vi "CMC-Random_Number_Alarms.vi"() -> ()   [LabVIEW 2010]
panel:
  out "Ok":bool
  out "Low Alarm":bool
  out "High Alarm":bool
  in  "Low Alarm":dbl=0.05 min=0.05 max=0.45
  in  "High Alarm":dbl=0.65 min=0.65 max=0.95 format="%#.2g"
  out "number(0 to 1)":dbl(slide) scale=0.0..1.0
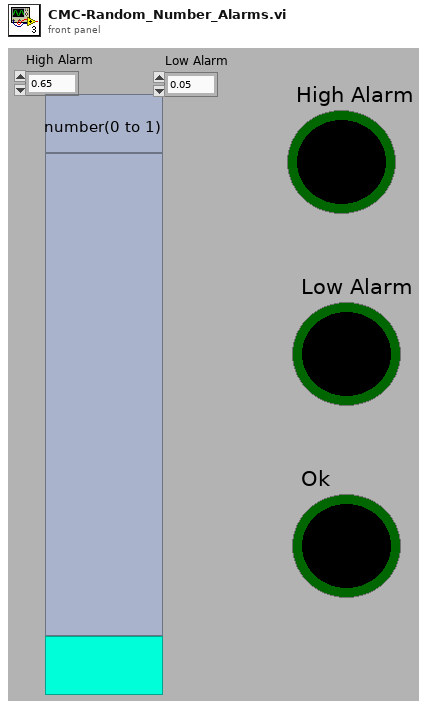
[diagram p1: front panel]
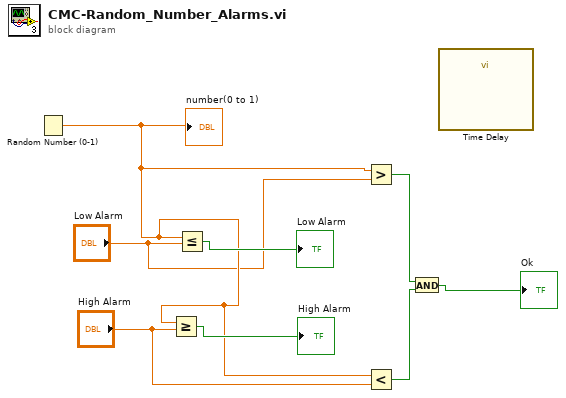
[diagram p0: block diagram]
diagram:
  n1 = Random Number (0-1)() -> (number: 0 to 1=w2:dbl)
  "number(0 to 1)" <- w2
  n2 = Greater Or Equal?(x=w2, y="High Alarm") -> (x >= y?=→"High Alarm":bool)
  n3 = Less Or Equal?(x=w2, y="Low Alarm") -> (x <= y?=→"Low Alarm":bool)
  n4 = Greater?(x=w2, y="Low Alarm") -> (0:w5:bool)
  n5 = Less?(x=w2, y="High Alarm") -> (x < y?=w4:bool)
  n6 = And(x=w5, y=w4) -> (x .and. y?=→"Ok":bool)
  n7 = call "Time Delay"() -> ()  [unwired: 11 in, 1 out]
